vi "Within Range of 20 Feet.vi"(11 "BUTTON":bool) -> (1 "Bottom RPM":dbl, 3 "Top RPM":dbl)   [LabVIEW 2019]
uses:
  <vilib>/Rock Robotics/Network Tables/NT Read Number.vi
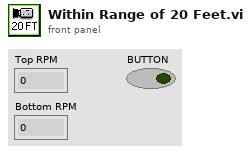
[diagram p1: front panel]
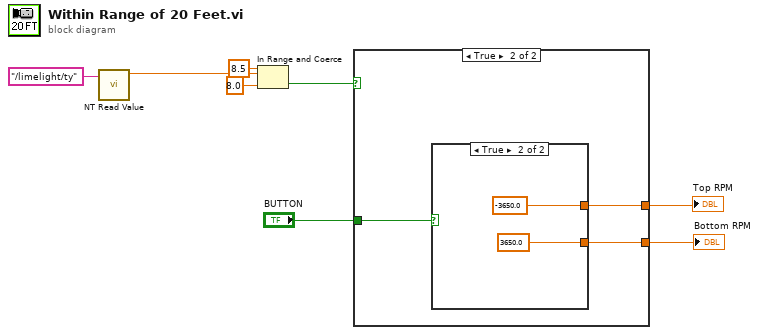
[diagram p0: block diagram]
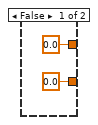
[diagram p2: hidden frame]
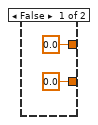
[diagram p3: hidden frame]
diagram:
  n1 = call-poly <vilib>:"NT Read Value.vi"("Name"="/limelight/ty") -> ("Numeric"=w4:dbl)  [unwired: 9 in, 1 out]
  n2 = In Range and Coerce(upper limit=8.5, x=w4, lower limit=8.0) -> (In Range?=w5:bool)  [unwired: 1 out]
  n3 = case shown="True" w5 {
    tunnel: "BUTTON" -> [_ w13]
    tunnel: [0.0 ("Top RPM") w12] -> w7
    tunnel: [0.0 ("Bottom RPM") w11] -> w8
    frame False {
    }
    frame True {
      n4 = case shown="True" w13 {
        tunnel: [0.0 ("Top RPM") -3650.0 ("Top RPM")] -> w12
        tunnel: [0.0 ("Bottom RPM") 3650.0 ("Bottom RPM")] -> w11
        frame False {
        }
        frame True {
        }
      }
    }
  }
  "Top RPM" <- w7
  "Bottom RPM" <- w8
